vi "medicaoIXV.vi"() -> ()   [LabVIEW 2012]
uses:
  <vilib>/Utility/file.llb/Write To Spreadsheet File (string).vi
  <vilib>/Utility/file.llb/Write To Spreadsheet File (DBL).vi
  <instrlib>/Agilent 6XXX Series/Agilent 6XXX Series.lvlib
panel:
  in  "Tab Control":enum32{"Entrada de dados", "Saída de dados"}(tab)
  out "ON/OFF":bool
  in  "Pontos":dbl
  in  "Tensão máxima":dbl
  in  "Nome da célula":string
  in  "Local":path
  in  "Delay(s)":dbl
  in  "Start":bool
  out "IXV":cluster{"Y":dbl[], "Y":dbl[]}[](graph)
  out "output voltage":dbl
  out "Tensao Atual":dbl
  out "Corrente Atual":dbl
  out "Ponto Atual":i32
  out "TABELA DE DADOS\nTensão(fonte)     Tensão                  Corrente            Pontos":dbl[][](array[numeric]) caption="all rows" format="%0.3f"
  in  "CorrenteGraph":dbl
  in  "error in (no error)":errorcluster
  out "error out":errorcluster
  in  "TensaoGraph":dbl
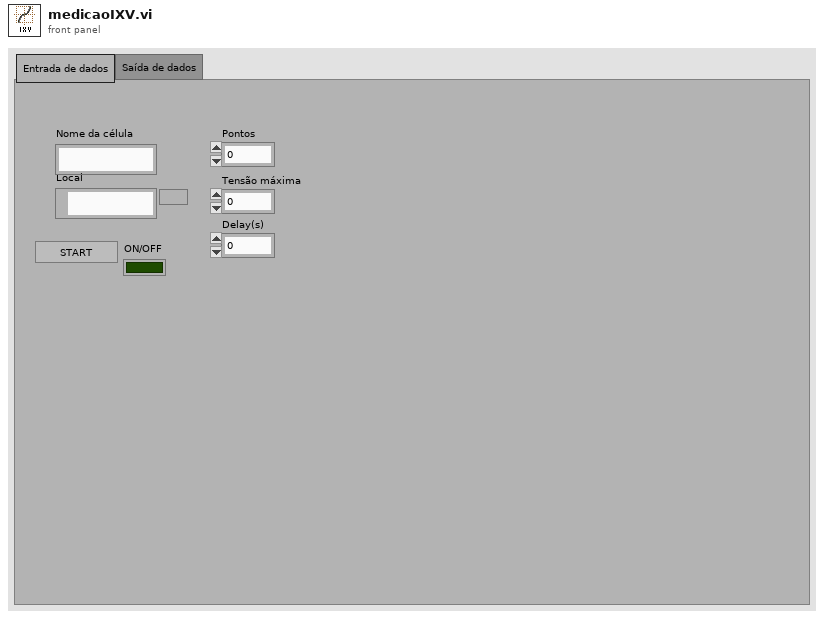
[diagram p1: front panel]
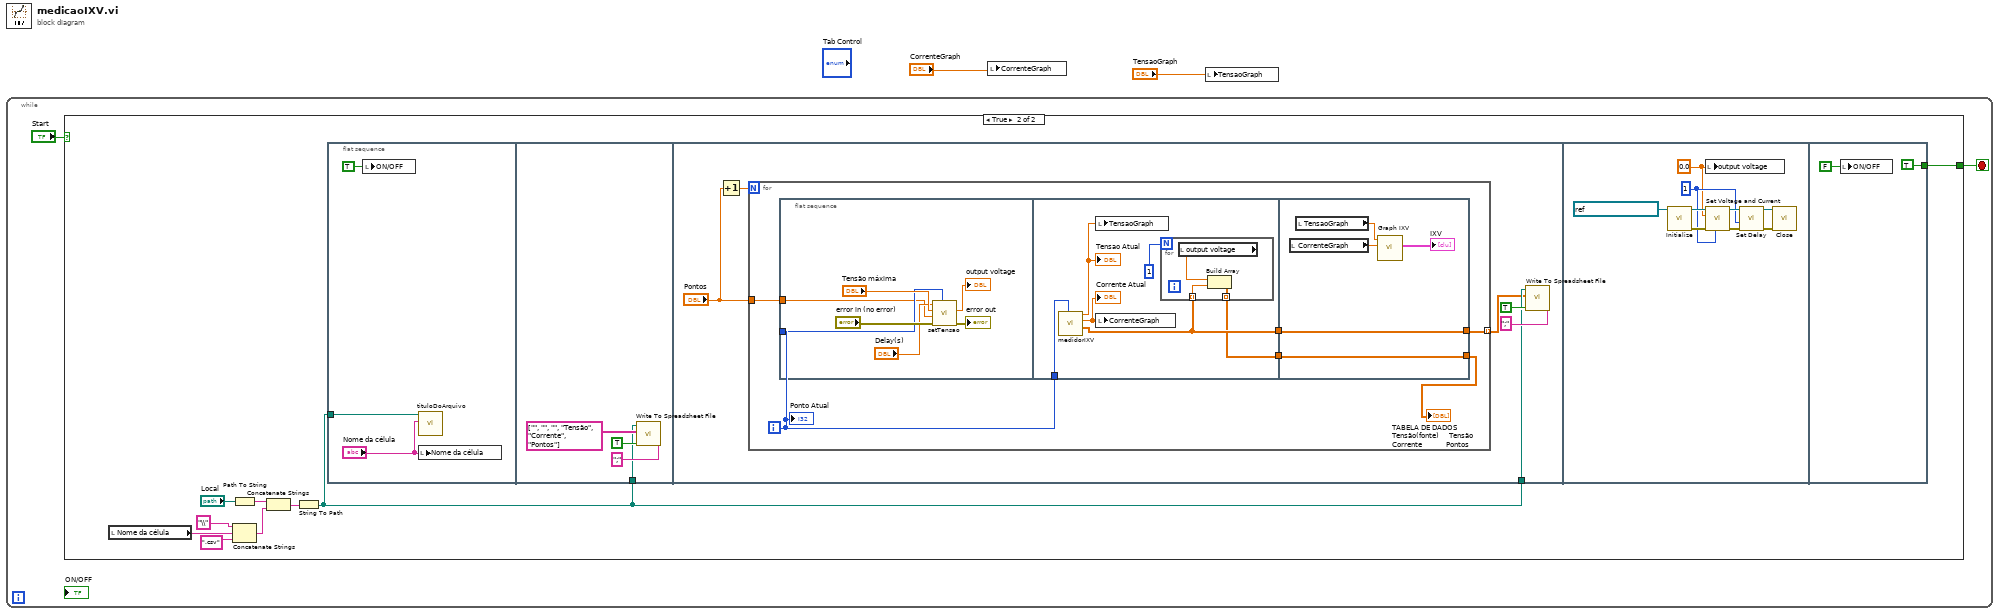
[diagram p0: block diagram]
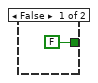
[diagram p2: hidden frame]
diagram:
  n1 = while {
    stop <- w3 stop-if-true
    n2 = case shown="True" "Start" {
      tunnel: [FALSE w8] -> w3
      frame False {
      }
      frame True {
        n3 = local read "Nome da célula"() -> (w9:string)
        n4 = Path To String(path="Local") -> (string=w13:string)
        n5 = Concatenate Strings("\\", w9, ".csv") -> (w14:string)
        n6 = Concatenate Strings(w13, w14) -> (w12:string)
        n7 = String To Path(string=w12) -> (path=w6:path)
        n8 = flat-sequence {
          tunnel: w6 -> [w16]
          tunnel: w6 -> [w18]
          tunnel: w6 -> [w25]
          tunnel: [TRUE] -> w8
          frame #0 {
            n9 = local write "ON/OFF"(TRUE ("ON/OFF")) -> ()
            n10 = call "tituloDoArquivo.vi"("Nome da célula"="Nome da célula", "file path (dialog if empty)"=w16) -> ()  [unwired: 10 in]
            n11 = local write "Nome da célula"("Nome da célula") -> ()
          }
          frame #1 {
            n12 = call-poly <vilib>:"Write To Spreadsheet File.vi"("delimiter (\\t)"=";" ("delimiter (\\t)"), "append to file? (new file:F)"=TRUE, "2D data"=string[][] [["", "", ""], ["Tensão", "Corrente", "Pontos"]], "file path (dialog if empty)"=w18) -> ()  [unwired: 4 in, 1 out]
          }
          frame #2 {
            n13 = Increment(x="Pontos") -> (x+1=w24:dbl)
            n14 = for {
              N: w24 -> [_]
              tunnel: [w31] -> w22 mode=indexing
              tunnel: "Pontos" -> [w33]
              i -> [w32]
              n15 = flat-sequence {
                tunnel: w33 -> [w36]
                tunnel: w32 -> [w37]
                tunnel: w32 -> [w46]
                tunnel: [w43] -> w30
                tunnel: [w42] -> w29
                tunnel: [w53] -> w28
                tunnel: [w54] -> w31
                tunnel: w30 -> [w54]
                tunnel: w29 -> [w53]
                frame #0 {
                  n16 = call "setTensao.vi"("Ponto"=w37, "error in (no error)"="error in (no error)", "Pontos"=w36, "Tensão máxima"="Tensão máxima", "delay(s)"="Delay(s)") -> ("error out"=→"error out":errorcluster, "output voltage"=→"output voltage":dbl)  [unwired: 5 in]
                }
                frame #1 {
                  n17 = call "medidorIXV.vi"("Ponto"=w46) -> ("Array"=w43:dbl[], "Corrente Atual"=w45:dbl, "Tensao Atual"=w44:dbl)  [unwired: 8 in]
                  "Corrente Atual" <- w45
                  "Tensao Atual" <- w44
                  n18 = local write "TensaoGraph"(w44) -> ()
                  n19 = local write "CorrenteGraph"(w45) -> ()
                  n20 = for {
                    N: 1 -> [_]
                    tunnel: w43 -> [w48] mode=indexing
                    tunnel: [w47] -> w42 mode=indexing
                    n21 = local read "output voltage"() -> (w49:dbl)
                    n22 = Build Array(w49, w48) -> (w47:dbl[])
                  }
                }
                frame #2 {
                  n23 = local read "CorrenteGraph"() -> (w50:dbl)
                  n24 = local read "TensaoGraph"() -> (w51:dbl)
                  n25 = call "Graph IXV"("Y Input"=w50, "X Input"=w51) -> ("XY Graph"=→"IXV":cluster{"Y":dbl[], "Y":dbl[]}[])  [unwired: 3 in, 6 out]
                }
              }
              "Ponto Atual" <- w32
              "TABELA DE DADOS\nTensão(fonte)     Tensão                  Corrente            Pontos" <- w28
            }
            n26 = call-poly <vilib>:"Write To Spreadsheet File.vi"("delimiter (\\t)"=";" ("delimiter (\\t)"), "append to file? (new file:F)"=TRUE, "2D data"=w22, "file path (dialog if empty)"=w25) -> ()  [unwired: 4 in, 1 out]
          }
          frame #3 {
            w55 = 0.0 ("voltage (0 V)")
            w58 = u8 1 ("channel (1)")
            n27 = call <instrlib>:"Initialize.vi"("VISA resource name"=refnum<visa-resource-name> "GPIB0::5::INSTR") -> ("error out"=w60:errorcluster, "VISA resource name out"=w59:refnum<visa-resource-name>)  [unwired: 9 in]
            n28 = local write "output voltage"(w55) -> ()
            n29 = call <instrlib>:"Set Voltage and Current.vi"("channel (1)"=w58, "error in (no error)"=w60, "voltage (0 V)"=w55, "VISA resource name"=w59) -> ("error out"=w61:errorcluster, "VISA resource name out"=w62:refnum<visa-resource-name>)  [unwired: 6 in]
            n30 = call <instrlib>:"Set Delay.vi"("error in (no error)"=w61, "channel (1)"=w58, "VISA resource name"=w62) -> ("error out"=w56:errorcluster, "VISA resource name out"=w57:refnum<visa-resource-name>)  [unwired: 7 in]
            n31 = call <instrlib>:"Close.vi"("error in (no error)"=w56, "VISA resource name"=w57) -> ()  [unwired: 9 in, 1 out]
          }
          frame #4 {
            n32 = local write "ON/OFF"(FALSE) -> ()
          }
        }
      }
    }
  }
  n33 = local write "CorrenteGraph"("CorrenteGraph") -> ()
  n34 = local write "TensaoGraph"("TensaoGraph") -> ()
